vi "Main 2.vi"() -> ()   [LabVIEW 2026]
uses:
  Desktop/industrial-machine-simulation/statemachine.ctl
  <vilib>/numeric/Random Number (Range) DBL.vi
panel:
  in  "EMERGENCY":bool
  out "Thermometer":dbl(slide)=22.025379166725855 scale=0.0..200.0
  out "You need product":bool=TRUE
  in  "PAUSE":bool
  in  "speed":i32(listbox)
  in  "RPM x1000":dbl(knob)=-1.0296070099394212 scale=0.0..10.0
  out "Enum":T1
  in  "Products":u16=50
  in  "Machine Start":bool
  in  "STOP":bool
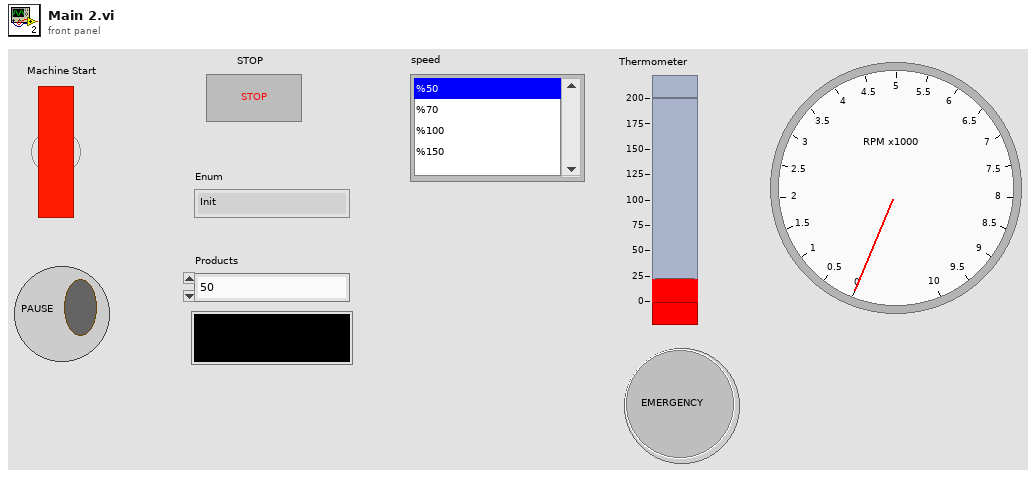
[diagram p1: front panel]
types:
  T1 = typedef "statemachine.ctl" = enum16{"Init", "Ready", "Running", "Paused", "Emergency"}
  T2 = cluster{"Products":u16, "RPM x1000":dbl, "speed":i32, "Thermometer":dbl, "EMERGENCY":bool}
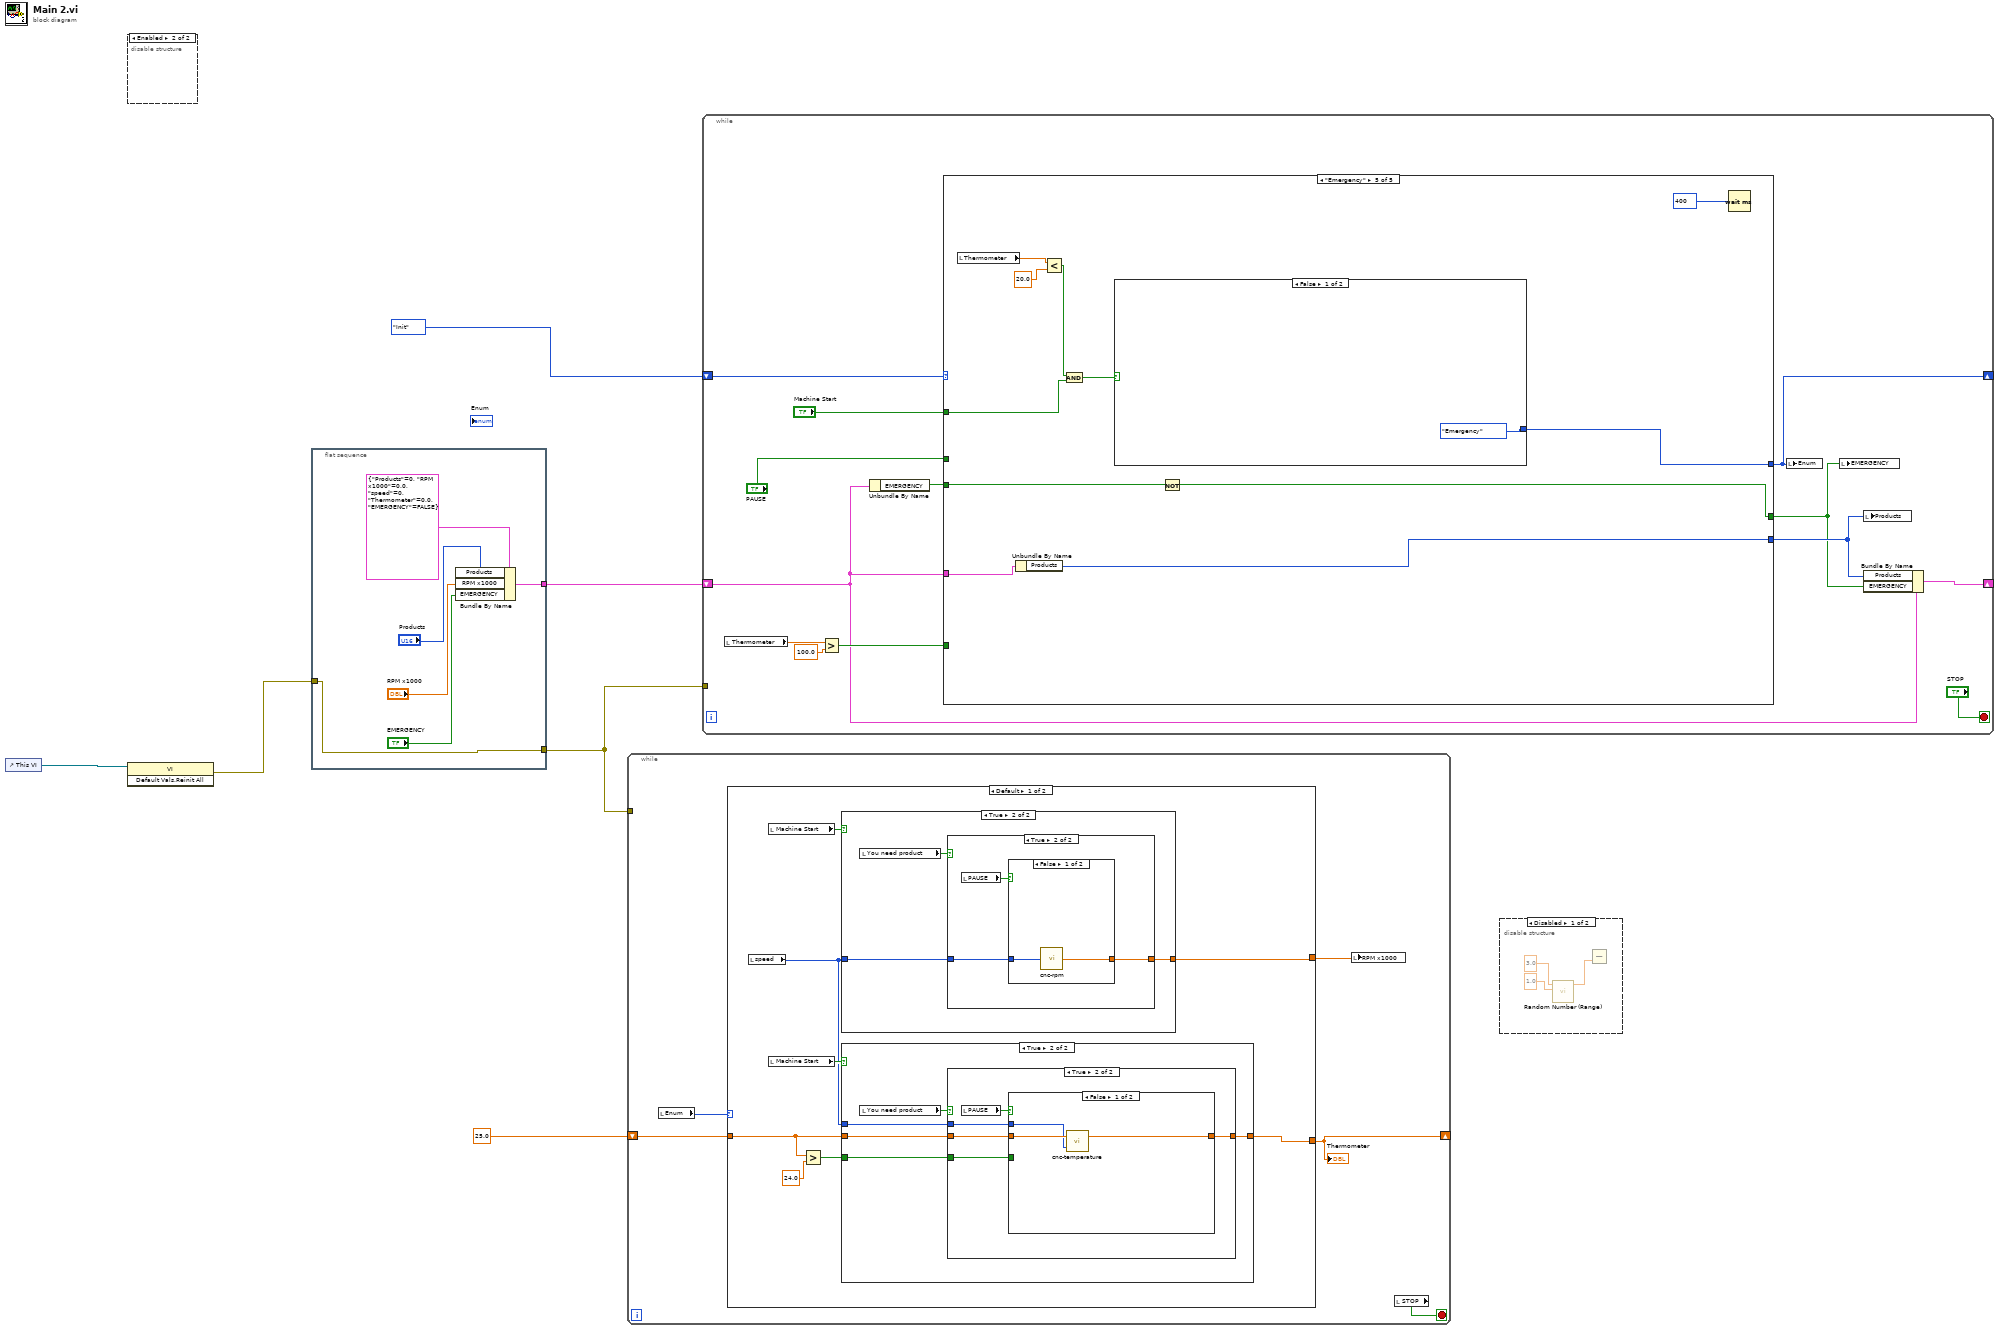
[diagram p0: block diagram]
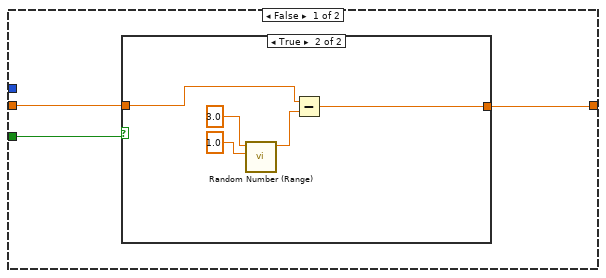
[diagram p3: hidden frame]
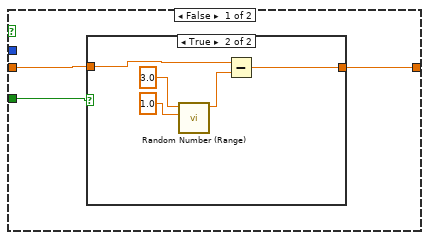
[diagram p5: hidden frame]
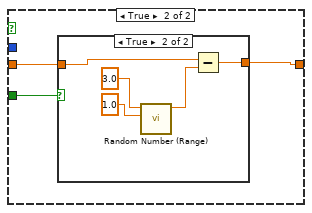
[diagram p7: hidden frame]
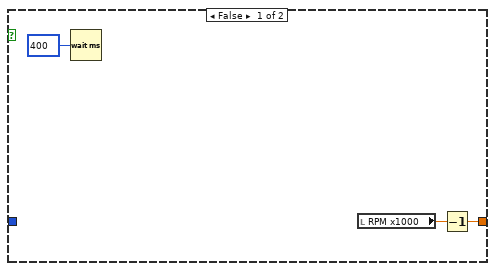
[diagram p9: hidden frame]
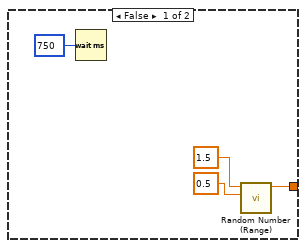
[diagram p10: hidden frame]
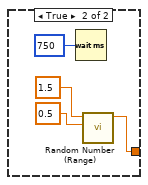
[diagram p11: hidden frame]
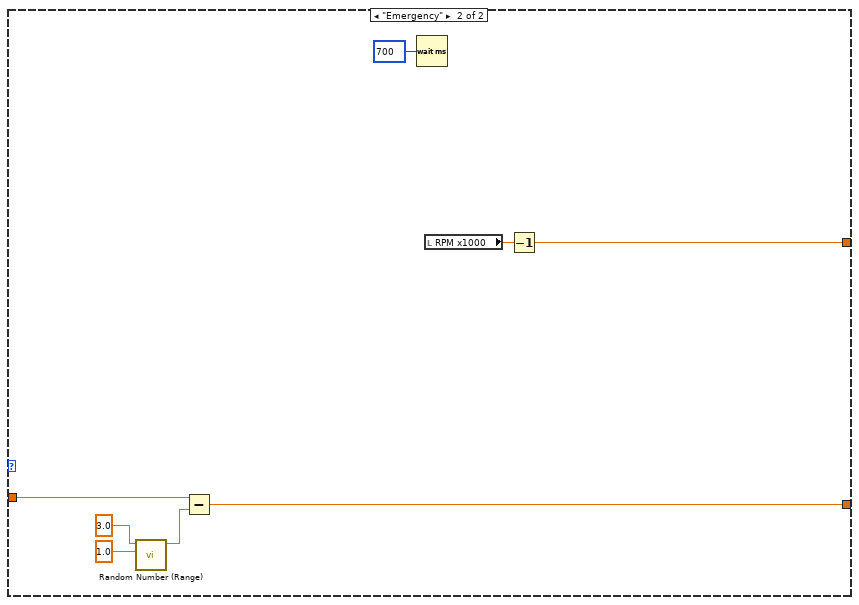
[diagram p12: hidden frame]
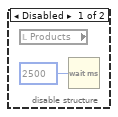
[diagram p13: hidden frame]
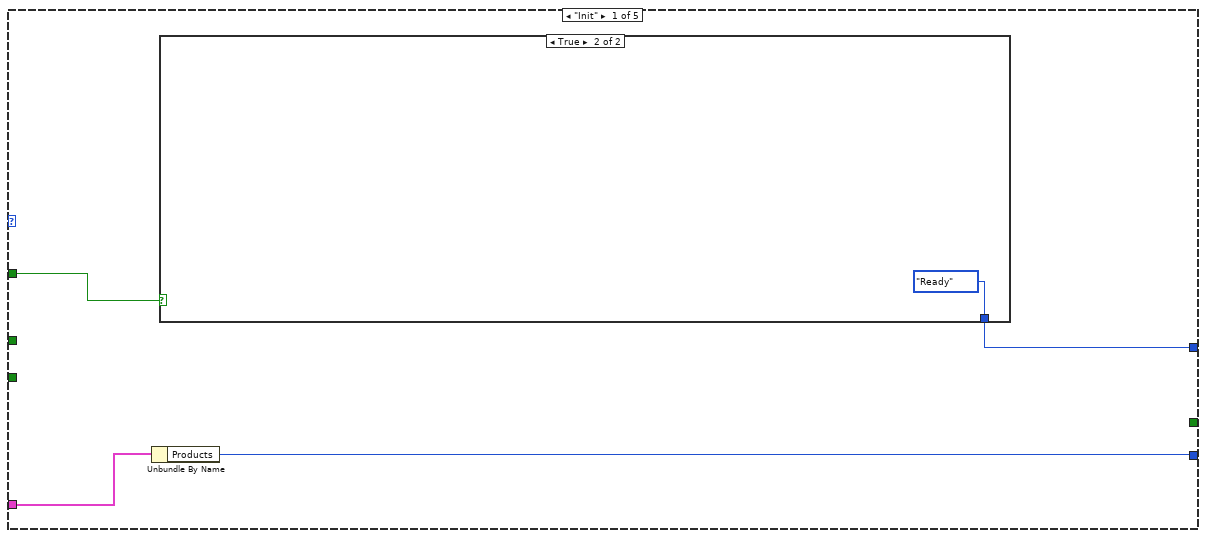
[diagram p14: hidden frame]
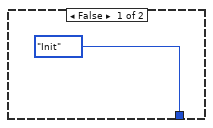
[diagram p15: hidden frame]
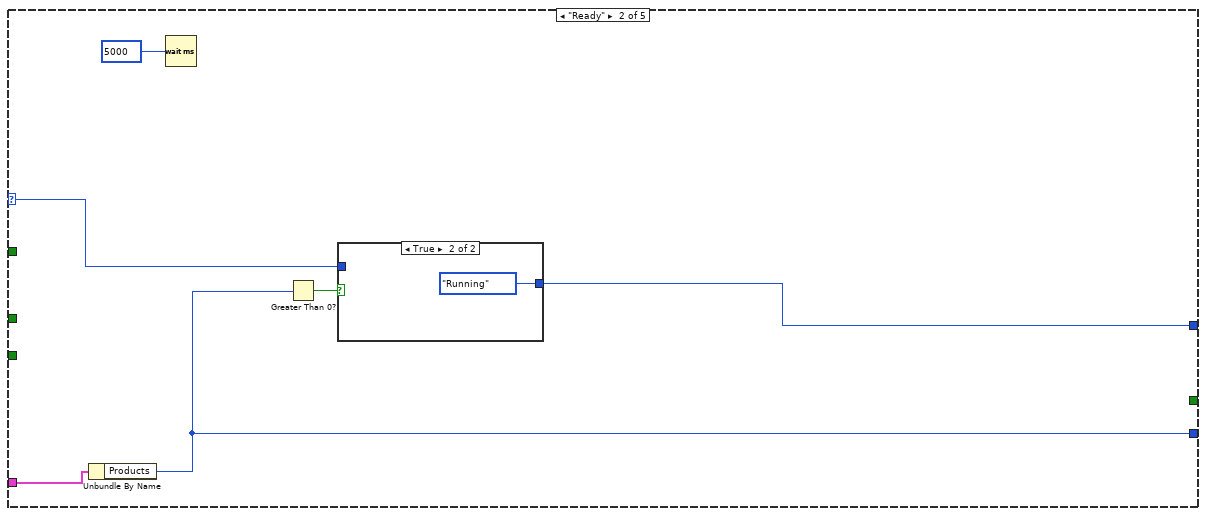
[diagram p16: hidden frame]
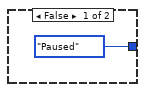
[diagram p17: hidden frame]
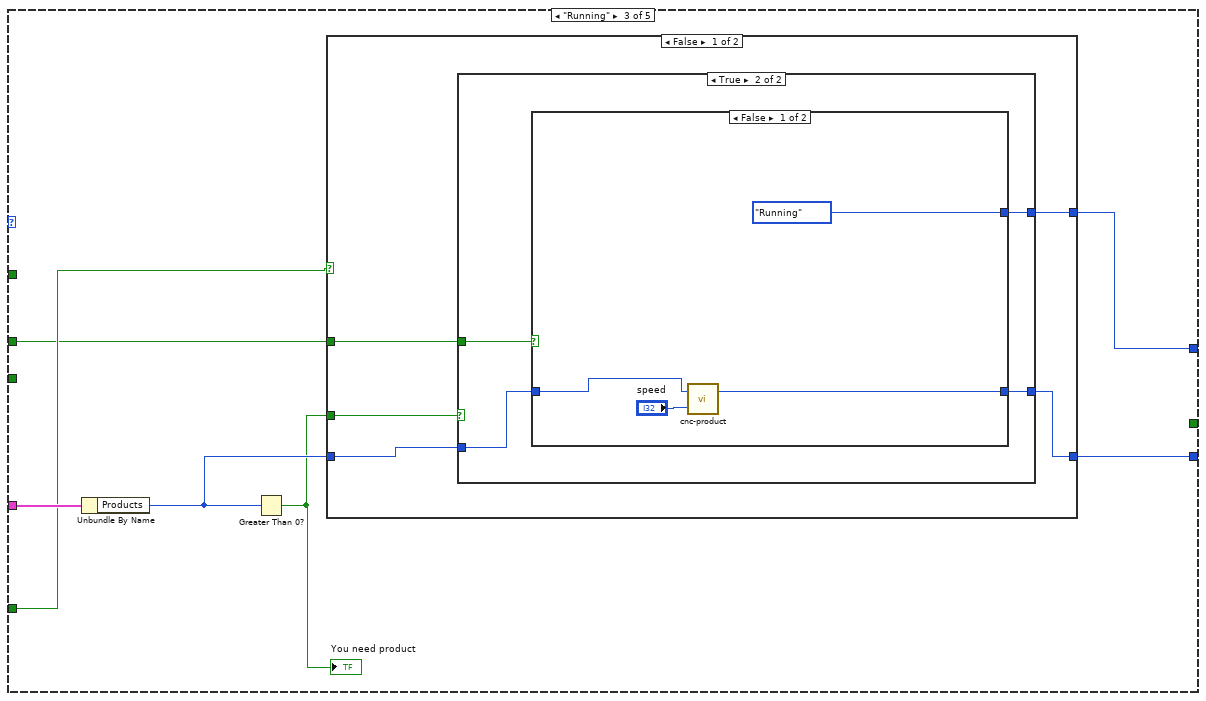
[diagram p18: hidden frame]
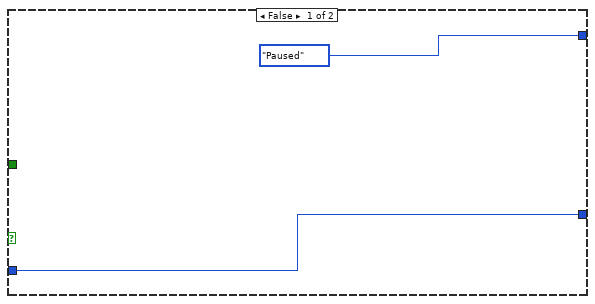
[diagram p19: hidden frame]
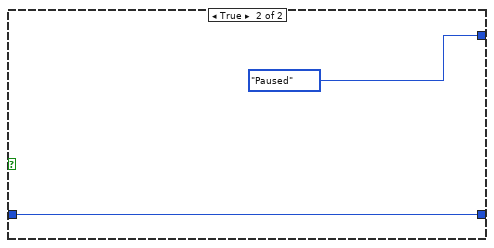
[diagram p20: hidden frame]
diagram:
  n1 = control-ref of="This VI"() -> (w3:refnum<vi>)
  n2 = disable-structure shown="Enabled" {
    frame Disabled {
      n3 = local read "Products"() -> ()  [unwired: 1 out]
      n4 = Wait (ms)(milliseconds to wait=u32 2500) -> ()  [unwired: 1 out]
    }
    frame Enabled {
    }
  }
  n5 = invoke class="VI" method="Default Vals.Reinit All"(reference=w3) -> (error out=w2:errorcluster)  [unwired: 2 in, 2 out]
  n6 = flat-sequence {
    tunnel: [w13] -> w6
    tunnel: w2 -> [w8]
    tunnel: [w8] -> w1
    frame #0 {
      n7 = Bundle By Name(cluster=T2 {"Products"=0, "RPM x1000"=0.0, "speed"=0, "Thermometer"=0.0, "EMERGENCY"=FALSE}, "Products"="Products", "RPM x1000"="RPM x1000", "EMERGENCY"="EMERGENCY") -> (w13:T2)
    }
  }
  n8 = while {
    shift-right: [w16] -> _
    shift-left: 25.0 ("Thermometer") -> [w17]
    tunnel: w1 -> [_]
    stop <- w18 stop-if-true
    n9 = local read "Enum"() -> (w14:T1)
    n10 = case shown="Default" w14 {
      tunnel: w17 -> [w20 w90]
      tunnel: [w23 w89] -> w16
      tunnel: [w19 w86] -> w15
      frame Default {
        n11 = local read "speed"() -> (w24:i32)
        n12 = local read "Machine Start"() -> (w26:bool)
        n13 = local read "Machine Start"() -> (w25:bool)
        n14 = Greater?(x=w20, y=24.0 ("Thermometer")) -> (0:w21:bool)
        n15 = case shown="True" w26 {
          tunnel: w24 -> [_ w72]
          tunnel: [w68 w71] -> w19
          frame False {
            n16 = Wait (ms)(milliseconds to wait=u32 400) -> ()  [unwired: 1 out]
            n17 = local read "RPM x1000"() -> (w69:dbl)
            n18 = Decrement(x=w69) -> (x-1=w68:dbl)
          }
          frame True {
            n19 = local read "You need product"() -> (w70:bool)
            n20 = case shown="True" w70 {
              tunnel: w72 -> [_ w78]
              tunnel: [w73 w77] -> w71
              frame False {
                n21 = Wait (ms)(milliseconds to wait=u32 750) -> ()  [unwired: 1 out]
                n22 = call-poly <vilib>:"Random Number (Range).vi"("lower bound (0)"=0.5, "upper bound (100)"=1.5) -> ("number"=w73:dbl)  [unwired: 9 in]
              }
              frame True {
                n23 = local read "PAUSE"() -> (w79:bool)
                n24 = case shown="False" w79 {
                  tunnel: w78 -> [w81 _]
                  tunnel: [w80 w83] -> w77
                  frame False {
                    n25 = call "cnc-rpm.vi"("speed in"=w81) -> ("rpm out"=w80:dbl)
                  }
                  frame True {
                    n26 = Wait (ms)(milliseconds to wait=u32 750) -> ()  [unwired: 1 out]
                    n27 = call-poly <vilib>:"Random Number (Range).vi"("lower bound (0)"=0.5, "upper bound (100)"=1.5) -> ("number"=w83:dbl)  [unwired: 9 in]
                  }
                }
              }
            }
          }
        }
        n28 = case shown="True" w25 {
          tunnel: w20 -> [w29 w39]
          tunnel: w24 -> [_ w38]
          tunnel: [w28 w37] -> w23
          tunnel: w21 -> [w27 w36]
          frame False {
            n29 = case shown="True" w27 {
              tunnel: w29 -> [w30 w32]
              tunnel: [w30 w31] -> w28
              frame False {
              }
              frame True {
                n30 = call-poly <vilib>:"Random Number (Range).vi"("lower bound (0)"=1.0, "upper bound (100)"=3.0) -> ("number"=w35:dbl)  [unwired: 9 in]
                n31 = Subtract(x=w32, y=w35) -> (x-y=w31:dbl)
              }
            }
          }
          frame True {
            n32 = local read "You need product"() -> (w40:bool)
            n33 = case shown="True" w40 {
              tunnel: w39 -> [w42 w53]
              tunnel: w38 -> [_ w52]
              tunnel: [w43 w51] -> w37
              tunnel: w36 -> [w41 w50]
              frame False {
                n34 = case shown="True" w41 {
                  tunnel: [w44 w46] -> w43
                  tunnel: w42 -> [w44 w45]
                  frame False {
                  }
                  frame True {
                    n35 = call-poly <vilib>:"Random Number (Range).vi"("lower bound (0)"=1.0, "upper bound (100)"=3.0) -> ("number"=w49:dbl)  [unwired: 9 in]
                    n36 = Subtract(x=w45, y=w49) -> (x-y=w46:dbl)
                  }
                }
              }
              frame True {
                n37 = local read "PAUSE"() -> (w54:bool)
                n38 = case shown="False" w54 {
                  tunnel: w53 -> [w57 w60]
                  tunnel: w52 -> [w56 _]
                  tunnel: [w55 w59] -> w51
                  tunnel: w50 -> [_ w58]
                  frame False {
                    n39 = call "cnc-temperature.vi"("speed in"=w56, "Temperature in"=w57) -> ("Temperature out"=w55:dbl)  [unwired: 1 in]
                  }
                  frame True {
                    n40 = case shown="True" w58 {
                      tunnel: w60 -> [w61 w63]
                      tunnel: [w61 w62] -> w59
                      frame False {
                      }
                      frame True {
                        n41 = call-poly <vilib>:"Random Number (Range).vi"("lower bound (0)"=1.0, "upper bound (100)"=3.0) -> ("number"=w64:dbl)  [unwired: 9 in]
                        n42 = Subtract(x=w63, y=w64) -> (x-y=w62:dbl)
                      }
                    }
                  }
                }
              }
            }
          }
        }
      }
      frame "Emergency" {
        n43 = call-poly <vilib>:"Random Number (Range).vi"("lower bound (0)"=1.0, "upper bound (100)"=3.0) -> ("number"=w93:dbl)  [unwired: 9 in]
        n44 = Subtract(x=w90, y=w93) -> (x-y=w89:dbl)
        n45 = Wait (ms)(milliseconds to wait=u32 700) -> ()  [unwired: 1 out]
        n46 = local read "RPM x1000"() -> (w88:dbl)
        n47 = Decrement(x=w88) -> (x-1=w86:dbl)
      }
    }
    "Thermometer" <- w16
    n48 = local write "RPM x1000"(w15) -> ()
    n49 = local read "STOP"() -> (w18:bool)
  }
  n50 = while {
    shift-right: [w104] -> _
    shift-left: statemachine."Init" ("Enum") -> [w105]
    shift-right: [w103] -> _
    shift-left: w6 -> [w96]
    tunnel: w1 -> [_]
    stop <- "STOP" stop-if-true
    n51 = local read "Thermometer"() -> (w97:dbl)
    n52 = Greater?(x=w97, y=100.0) -> (0:w98:bool)
    n53 = Unbundle By Name(w96) -> ("EMERGENCY"=w94:bool)
    n54 = case shown="\"Emergency\"" w105 {
      selector: w105 -> [_ w117 _ _ _]
      tunnel: [w108 w118 w127 w151 w165] -> w104
      tunnel: [w110 w114 w126 w153 w166] -> w102
      tunnel: "Machine Start" -> [w109 _ _ _ w163]
      tunnel: "PAUSE" -> [_ _ w121 w152 _]
      tunnel: w96 -> [w107 w113 w125 w149 w164]
      tunnel: w98 -> [_ _ w123 _ _]
      tunnel: [_ _ _ _ w157] -> w95
      tunnel: w94 -> [_ _ _ _ w158]
      frame "Init" {
        n55 = Unbundle By Name(w107) -> ("Products"=w110:u16)
        n56 = case shown="True" w109 {
          tunnel: [statemachine."Init" ("Enum") statemachine."Ready" ("Enum")] -> w108
          frame False {
          }
          frame True {
          }
        }
      }
      frame "Ready" {
        n57 = Unbundle By Name(w113) -> ("Products"=w114:u16)
        n58 = Wait (ms)(milliseconds to wait=u32 5000) -> ()  [unwired: 1 out]
        n59 = Greater Than 0?(x=w114) -> (x > 0?=w116:bool)
        n60 = case shown="True" w116 {
          tunnel: [statemachine."Paused" ("Enum") statemachine."Running" ("Enum")] -> w118
          tunnel: w117 -> [_ _]
          frame False {
          }
          frame True {
          }
        }
      }
      frame "Running" {
        n61 = Unbundle By Name(w125) -> ("Products"=w124:u16)
        n62 = Greater Than 0?(x=w124) -> (x > 0?=w122:bool)
        "You need product" <- w122
        n63 = case shown="False" w123 {
          tunnel: [w131 statemachine."Emergency" ("Enum")] -> w127
          tunnel: [w132 w147] -> w126
          tunnel: w124 -> [w130 w147]
          tunnel: w122 -> [w129 _]
          tunnel: w121 -> [w128 _]
          frame False {
            n64 = case shown="True" w129 {
              tunnel: [w134 w138] -> w132
              tunnel: [statemachine."Paused" ("Enum") w137] -> w131
              tunnel: w130 -> [w134 w136]
              tunnel: w128 -> [_ w135]
              frame False {
              }
              frame True {
                n65 = case shown="False" w135 {
                  tunnel: [w142 w144] -> w138
                  tunnel: [statemachine."Running" ("Enum") statemachine."Paused" ("Enum")] -> w137
                  tunnel: w136 -> [w140 w144]
                  frame False {
                    n66 = call "cnc-product.vi"("speed in"="speed", "Products in"=w140) -> ("Products out"=w142:u16)  [unwired: 1 in]
                  }
                  frame True {
                  }
                }
              }
            }
          }
          frame True {
            n67 = Wait (ms)(milliseconds to wait=u32 400) -> ()  [unwired: 1 out]
            n68 = local write "EMERGENCY"(TRUE ("EMERGENCY")) -> ()
          }
        }
      }
      frame "Paused" {
        n69 = case shown="False" w152 {
          tunnel: [statemachine."Running" ("Enum") statemachine."Paused" ("Enum")] -> w151
          frame False {
          }
          frame True {
          }
        }
        n70 = Wait (ms)(milliseconds to wait=u32 750) -> ()  [unwired: 1 out]
        n71 = Unbundle By Name(w149) -> ("Products"=w153:u16)
      }
      frame "Emergency" {
        n72 = local read "Thermometer"() -> (w161:dbl)
        n73 = Unbundle By Name(w164) -> ("Products"=w166:u16)
        n74 = Less?(x=w161, y=20.0) -> (x < y?=w159:bool)
        n75 = And(x=w159, y=w163) -> (x .and. y?=w162:bool)
        n76 = case shown="False" w162 {
          tunnel: [statemachine."Emergency" ("Enum") statemachine."Running" ("Enum")] -> w165
          frame False {
          }
          frame True {
          }
        }
        n77 = Not(x=w158) -> (.not. x?=w157:bool)
        n78 = Wait (ms)(milliseconds to wait=u32 400) -> ()  [unwired: 1 out]
      }
    }
    n79 = local write "Enum"(w104) -> ()
    n80 = local write "EMERGENCY"(w95) -> ()
    n81 = local write "Products"(w102) -> ()
    n82 = Bundle By Name(cluster=w96, "Products"=w102, "EMERGENCY"=w95) -> (w103:T2)
  }
  n83 = disable-structure shown="Disabled" {
    frame Disabled {
      n84 = call-poly <vilib>:"Random Number (Range).vi"("lower bound (0)"=1.0, "upper bound (100)"=3.0) -> ("number"=w172:dbl)  [unwired: 9 in]
      n85 = Subtract(y=w172) -> (x=w171:dbl)  [unwired: 1 out]
    }
    frame Enabled {
    }
  }
